vi "control_lasers_and_SMs_TIMING_TRUNCATED_LOOPS_ADD_ICC4C.vi"() -> ()   [LabVIEW 2021]
uses:
  <vilib>/DAQmx/write.llb/DAQmx Write (Analog 1D DBL NChan 1Samp).vi
  <vilib>/DAQmx/create/channels.llb/DAQmx Create Channel (AO-Voltage-Basic).vi
  <vilib>/DAQmx/miscellaneous.llb/DAQmx Fill In Error Info.vi
panel:
  in  "ICC4C 3 IV (0-10V)":dbl
  in  "ICC4C 2 IV (0-10V)":dbl
  in  "ICC4C 1 IV (0-10V)":dbl
  in  "ICC4C 0 IV (0-10V)":dbl
  in  "ICC4C 3 III (0-10V)":dbl
  in  "ICC4C 2 III (0-10V)":dbl
  in  "ICC4C 1 III (0-10V)":dbl
  in  "ICC4C 0 III (0-10V)":dbl
  in  "ICC4C 3 II (0-10V)":dbl
  in  "ICC4C 2 II (0-10V)":dbl
  in  "ICC4C 1 II (0-10V)":dbl
  in  "ICC4C 0 II (0-10V)":dbl
  in  "ICC4C 3 (0-10V)":dbl
  in  "ICC4C 2 (0-10V)":dbl
  in  "ICC4C 1 (0-10V)":dbl
  in  "ICC4C 0 (0-10V)":dbl
  in  "X2 (-10-10V) IV":dbl
  in  "Y2 (-10-10V) IV":dbl
  in  "X2 (-10-10V) III":dbl
  in  "Y2 (-10-10V) III":dbl
  in  "X2 (-10-10V) II":dbl
  in  "Y2 (-10-10V) II":dbl
  in  "Y2 (-10-10V)":dbl
  in  "X2 (-10-10V)":dbl
  in  "Continue Cycle?":bool
  out "Full Cycles":i32
  in  "Phase IV Duration (sec)":dbl=10.0 format="%.2f"
  in  "445 (0-10v) IV":dbl
  in  "488 (0-10v) IV":dbl
  in  "514 (0-10v) IV":dbl
  in  "561 (0-10v) IV":dbl
  in  "Blanking (0-10v) IV":dbl=10.0
  in  "X1 (-10-10V) IV":dbl
  in  "Y1 (-10-10V) IV":dbl
  out "Phase IV Iterations":i32
  in  "Phase III Duration (sec)":dbl=10.0 format="%.2f"
  in  "Phase II Duration (sec)":dbl=10.0 format="%.2f"
  in  "445 (0-10v) III":dbl
  in  "488 (0-10v) III":dbl
  in  "514 (0-10v) III":dbl
  in  "561 (0-10v) III":dbl
  in  "Blanking (0-10v) III":dbl=10.0
  in  "X1 (-10-10V) III":dbl
  in  "Y1 (-10-10V) III":dbl
  out "Phase III Iterations":i32
  in  "445 (0-10v) II":dbl
  in  "488 (0-10v) II":dbl
  in  "514 (0-10v) II":dbl
  in  "561 (0-10v) II":dbl
  in  "Blanking (0-10v) II":dbl=10.0
  in  "X1 (-10-10V) II":dbl
  in  "Y1 (-10-10V) II":dbl
  out "Phase II Iterations":i32
  out "Phase I Iterations":i32
  in  "Phase I Duration (sec)":dbl=10.0 format="%.2f"
  in  "Y1 (-10-10V)":dbl
  in  "X1 (-10-10V)":dbl
  in  "Blanking (0-10v)":dbl=10.0
  in  "561 (0-10v)":dbl
  in  "514 (0-10v)":dbl
  in  "488 (0-10v)":dbl
  in  "445 (0-10v)":dbl
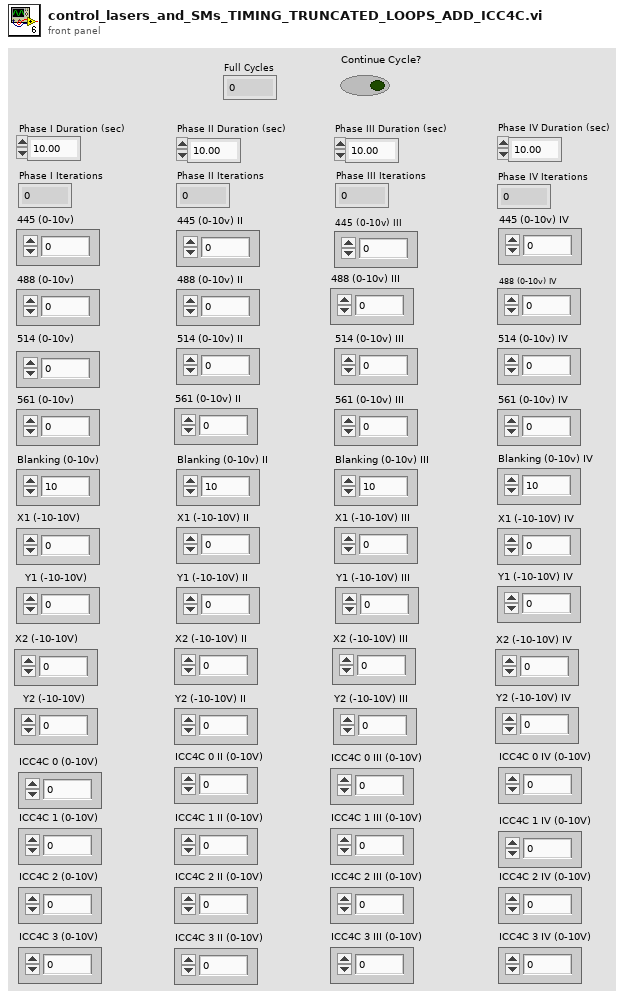
[diagram p1: front panel]
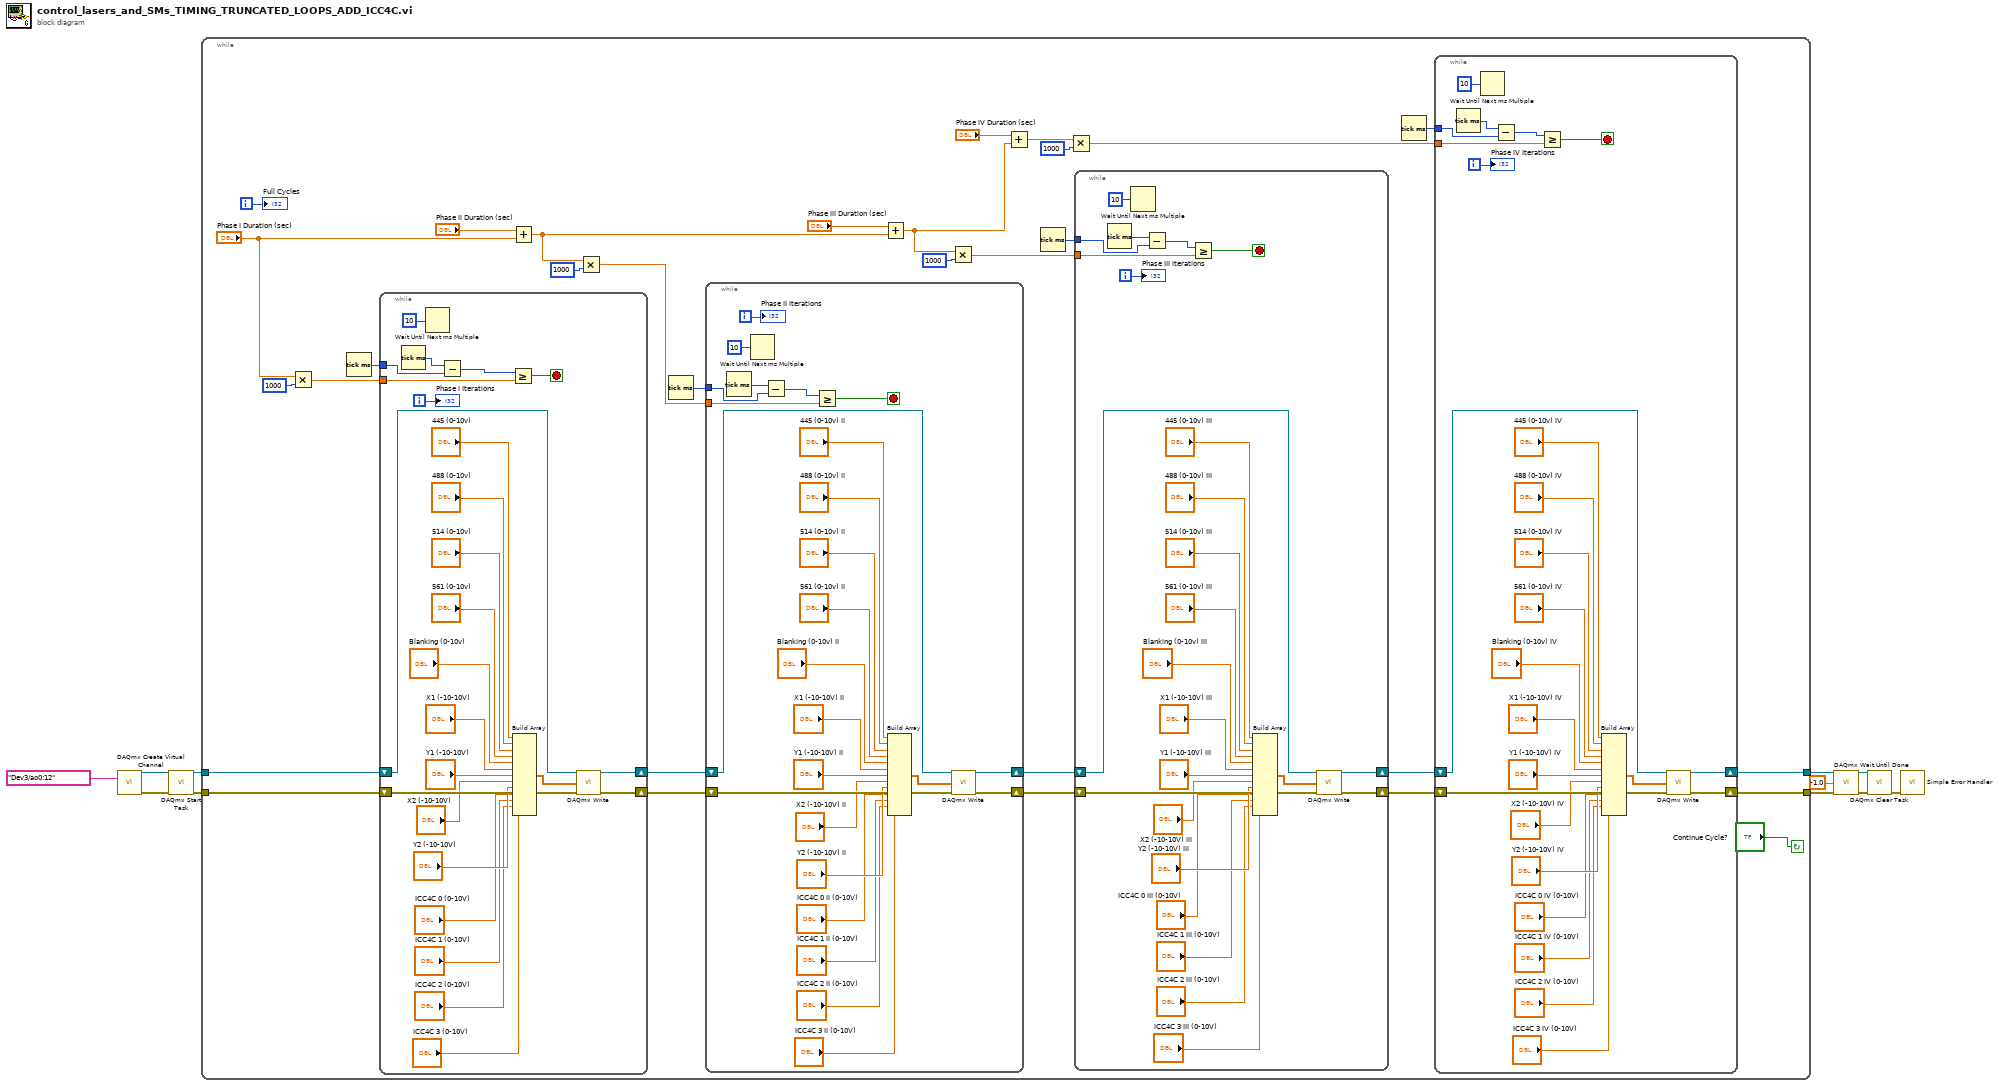
[diagram p0: block diagram]
diagram:
  n1 = call-poly <vilib>:"DAQmx Create Virtual Channel.vi"("physical channels"=tag "Dev3/ao0:12") -> ("task out"=w4:refnum<k21>, "error out"=w3:errorcluster)  [unwired: 13 in]
  n2 = call <vilib>:"DAQmx Start Task.vi"("task/channels in"=w4, "error in"=w3) -> ("task out"=w2:refnum<k21>, "error out"=w1:errorcluster)  [unwired: 12 in]
  n3 = while {
    tunnel: [w19] -> w7
    tunnel: [w18] -> w6
    tunnel: w2 -> [w14]
    tunnel: w1 -> [w13]
    i -> [w15]
    stop <- "Continue Cycle?" continue-if-true
    n4 = Multiply(x="Phase I Duration (sec)", y=1000) -> (x*y=w40:dbl)
    n5 = Tick Count (ms)() -> (millisecond timer value=w41:u32)
    n6 = while {
      shift-right: [w115] -> w33
      shift-left: w14 -> [w117]
      shift-right: [w114] -> w32
      shift-left: w13 -> [w116]
      tunnel: w41 -> [w104]
      tunnel: w40 -> [w100]
      i -> [w105]
      stop <- w101 stop-if-true
      n7 = Tick Count (ms)() -> (millisecond timer value=w103:u32)
      n8 = Wait Until Next ms Multiple(millisecond multiple=10) -> ()  [unwired: 1 out]
      n9 = Subtract(x=w103, y=w104) -> (x-y=w102:u32)
      n10 = Greater Or Equal?(x=w102, y=w100) -> (x >= y?=w101:bool)
      n11 = Build Array("445 (0-10v)", "488 (0-10v)", "514 (0-10v)", "561 (0-10v)", "Blanking (0-10v)", "X1 (-10-10V)", "Y1 (-10-10V)", "X2 (-10-10V)", "Y2 (-10-10V)", "ICC4C 0 (0-10V)", "ICC4C 1 (0-10V)", "ICC4C 2 (0-10V)", "ICC4C 3 (0-10V)") -> (w113:dbl[])
      n12 = call-poly <vilib>:"DAQmx Write.vi"("task/channels in"=w117, "data"=w113, "error in"=w116) -> ("task out"=w115:refnum<k21>, "error out"=w114:errorcluster)  [unwired: 10 in, 1 out]
      "Phase I Iterations" <- w105
    }
    n13 = Add(x="Phase II Duration (sec)", y="Phase I Duration (sec)") -> (x+y=w27:dbl)
    n14 = Multiply(x=w27, y=1000) -> (x*y=w37:dbl)
    n15 = Tick Count (ms)() -> (millisecond timer value=w38:u32)
    n16 = while {
      shift-right: [w90] -> w30
      shift-left: w33 -> [w92]
      shift-right: [w89] -> w31
      shift-left: w32 -> [w91]
      tunnel: w38 -> [w79]
      tunnel: w37 -> [w75]
      i -> [w80]
      stop <- w76 stop-if-true
      n17 = Tick Count (ms)() -> (millisecond timer value=w78:u32)
      n18 = Wait Until Next ms Multiple(millisecond multiple=10) -> ()  [unwired: 1 out]
      n19 = Subtract(x=w78, y=w79) -> (x-y=w77:u32)
      n20 = Greater Or Equal?(x=w77, y=w75) -> (x >= y?=w76:bool)
      n21 = Build Array("445 (0-10v) II", "488 (0-10v) II", "514 (0-10v) II", "561 (0-10v) II", "Blanking (0-10v) II", "X1 (-10-10V) II", "Y1 (-10-10V) II", "X2 (-10-10V) II", "Y2 (-10-10V) II", "ICC4C 0 II (0-10V)", "ICC4C 1 II (0-10V)", "ICC4C 2 II (0-10V)", "ICC4C 3 II (0-10V)") -> (w88:dbl[])
      n22 = call-poly <vilib>:"DAQmx Write.vi"("task/channels in"=w92, "data"=w88, "error in"=w91) -> ("task out"=w90:refnum<k21>, "error out"=w89:errorcluster)  [unwired: 10 in, 1 out]
      "Phase II Iterations" <- w80
    }
    n23 = Add(x="Phase III Duration (sec)", y=w27) -> (x+y=w24:dbl)
    n24 = Multiply(x=w24, y=1000) -> (x*y=w34:dbl)
    n25 = Add(x="Phase IV Duration (sec)", y=w24) -> (x+y=w23:dbl)
    n26 = Tick Count (ms)() -> (millisecond timer value=w35:u32)
    n27 = Multiply(x=w23, y=1000) -> (x*y=w25:dbl)
    n28 = while {
      shift-right: [w65] -> w21
      shift-left: w30 -> [w67]
      shift-right: [w64] -> w20
      shift-left: w31 -> [w66]
      tunnel: w35 -> [w54]
      tunnel: w34 -> [w50]
      i -> [w55]
      stop <- w51 stop-if-true
      n29 = Tick Count (ms)() -> (millisecond timer value=w53:u32)
      n30 = Wait Until Next ms Multiple(millisecond multiple=10) -> ()  [unwired: 1 out]
      n31 = Subtract(x=w53, y=w54) -> (x-y=w52:u32)
      n32 = Greater Or Equal?(x=w52, y=w50) -> (x >= y?=w51:bool)
      n33 = Build Array("445 (0-10v) III", "488 (0-10v) III", "514 (0-10v) III", "561 (0-10v) III", "Blanking (0-10v) III", "X1 (-10-10V) III", "Y1 (-10-10V) III", "X2 (-10-10V) III", "Y2 (-10-10V) III", "ICC4C 0 III (0-10V)", "ICC4C 1 III (0-10V)", "ICC4C 2 III (0-10V)", "ICC4C 3 III (0-10V)") -> (w63:dbl[])
      n34 = call-poly <vilib>:"DAQmx Write.vi"("task/channels in"=w67, "data"=w63, "error in"=w66) -> ("task out"=w65:refnum<k21>, "error out"=w64:errorcluster)  [unwired: 10 in, 1 out]
      "Phase III Iterations" <- w55
    }
    n35 = Tick Count (ms)() -> (millisecond timer value=w16:u32)
    n36 = while {
      shift-right: [w140] -> w19
      shift-left: w21 -> [w142]
      shift-right: [w139] -> w18
      shift-left: w20 -> [w141]
      tunnel: w16 -> [w129]
      tunnel: w25 -> [w125]
      i -> [w130]
      stop <- w126 stop-if-true
      n37 = Tick Count (ms)() -> (millisecond timer value=w128:u32)
      n38 = Wait Until Next ms Multiple(millisecond multiple=10) -> ()  [unwired: 1 out]
      n39 = Subtract(x=w128, y=w129) -> (x-y=w127:u32)
      n40 = Greater Or Equal?(x=w127, y=w125) -> (x >= y?=w126:bool)
      n41 = Build Array("445 (0-10v) IV", "488 (0-10v) IV", "514 (0-10v) IV", "561 (0-10v) IV", "Blanking (0-10v) IV", "X1 (-10-10V) IV", "Y1 (-10-10V) IV", "X2 (-10-10V) IV", "Y2 (-10-10V) IV", "ICC4C 0 IV (0-10V)", "ICC4C 1 IV (0-10V)", "ICC4C 2 IV (0-10V)", "ICC4C 3 IV (0-10V)") -> (w138:dbl[])
      n42 = call-poly <vilib>:"DAQmx Write.vi"("task/channels in"=w142, "data"=w138, "error in"=w141) -> ("task out"=w140:refnum<k21>, "error out"=w139:errorcluster)  [unwired: 10 in, 1 out]
      "Phase IV Iterations" <- w130
    }
    "Full Cycles" <- w15
  }
  n43 = call <vilib>:"DAQmx Wait Until Done.vi"("task/channels in"=w7, "timeout (sec)"=-1.0, "error in"=w6) -> ("task out"=w10:refnum<k21>, "error out"=w9:errorcluster)  [unwired: 11 in]
  n44 = call <vilib>:"DAQmx Clear Task.vi"("task in"=w10, "error in"=w9) -> ("error out"=w11:errorcluster)  [unwired: 13 in]
  n45 = call <vilib>:"Simple Error Handler.vi"("error in (no error)"=w11) -> ()  [unwired: 4 in, 5 out]
